vi "Scalar Channels_Various Types_FPGA_VI.vi"() -> ()   [LabVIEW 2018]
uses:
  D:/GitBranches/niveristand-fpga-addon-custom-device-1/Source/Submodules/Source/Types/Sine.Generate.Settings.ctl
  <vilib>/rvi/Emulation/niFpgaGetClockAttributes.vi
  <vilib>/rvi/Emulation/niFpgaSctlEmulationGetInTimedLoop.vi
  <vilib>/rvi/Emulation/niFpgaEmulationReportErrorSimple.vi
  <vilib>/rvi/Emulation/niFpgaCriticalErrorInLSC.vi
  D:/GitBranches/niveristand-fpga-addon-custom-device-1/Source/Submodules/Source/Speciality FPGA IO.lvlib
panel:
  out "3.5 Signed Indicator":fxp<+/-,4,3>=3.5
  out "1.5 Unsigned Indicator":fxp<+,3,2>=1.5
  out "U8 Indicator":u8
  in  "IO 2":T1={"AMP"=5.0, "OFFSET"=8.0, "PERIODS/TICKS"=0.49999999930150807}
  in  "IO":T1={"AMP"=3.0, "OFFSET"=4.0, "PERIODS/TICKS"=0.9999999997671694}
  in  "SGL":sgl=15.45
  in  "I32":i32=-150000
  in  "U32":u32=4294965496
  in  "I16":i16=-1800
  in  "U16":u16=950
  in  "I8":i8=-4
  in  "U8":u8=9
  in  "-1.75":fxp<+/-,8,2>=-1.75
  in  "3.5 Signed":fxp<+/-,4,3>=3.5
  in  "1.5 Unsigned":fxp<+,3,2>=1.5
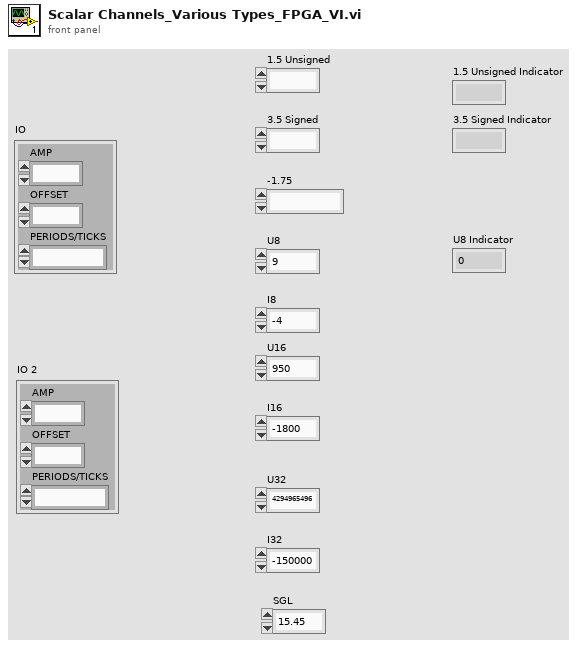
[diagram p1: front panel]
types:
  T1 = typedef "Speciality FPGA IO.lvlib/Sine.Generate.Settings.ctl" = cluster{"AMP":fxp<+/-,32,8>, "OFFSET":fxp<+/-,32,8>, "PERIODS/TICKS":fxp<+,32,0>}
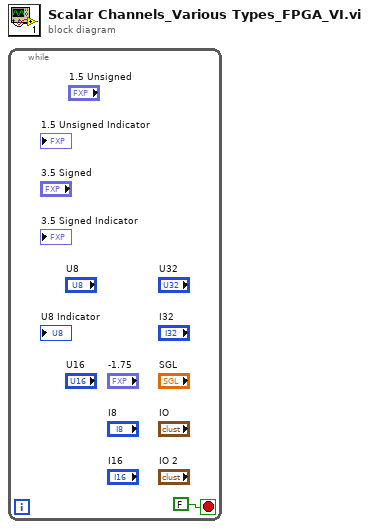
[diagram p0: block diagram]
diagram:
  n1 = while {
    stop <- FALSE stop-if-true
  }
